vi "Drive Controller.vi"(8 "error in":errorcluster) -> ()   [LabVIEW 2017]
doc: "This VI executes continuously carrying out the current operation and responding to updates or new operation requests. It will often contain the timing or control code that is difficult to place directly in TeleOp. This VI generally opens all sensors and motors and isolates the rest of the robot code from knowing implementation details of how the operations are carried out."
uses:
  <vilib>/Rock Robotics/WPI/Framework/Completion Status.ctl
  Drive Setpoints.ctl
  Drive Operations.ctl
  <vilib>/Rock Robotics/WPI/SafetyOutput/WPI_SafetyOutputConfigMenu.ctl
  Motor Settings.ctl
  <vilib>/Rock Robotics/SystemInterfaces/DIO/FPGA_DIOPWMChannel.ctl
  <vilib>/Rock Robotics/SystemInterfaces/DIO/FPGA_DIOChannel.ctl
  <vilib>/Rock Robotics/WPI/Counter/WPI_CounterDigitalInputToDigitalSource.vi
  <vilib>/Rock Robotics/Network Tables/NT Write Boolean.vi
panel:
  in  "Interactive Values":T1
  in  "Buttons":cluster{"Execute Cmd":bool, "Abort Cmd":bool}
  out "Command Timing":cluster{"Start Time (ms)":u32, "Iterations":i32}
  out "Status":T3
  out "Setpoints":T4(graph)
  out "Current\nCmd":string
  # "Tip: The graph shows the motor setpoints. It may also be helpful to observe inputs and sensor values.\nYou may also want to display tuning or debugging controls."
  # "Interactive Command: You may fill in the settings for a command\nand schedule it with the Execute button. You can observe and abort\nany command while fine tuning the code for the controller."
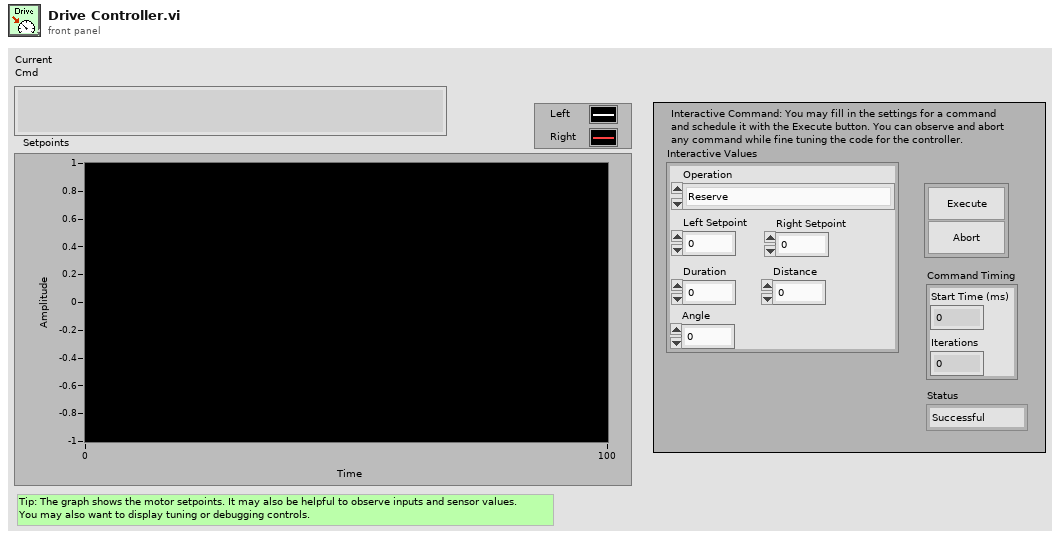
[diagram p1: front panel]
types:
  T1 = typedef "Drive Setpoints.ctl" = cluster{"Operation":T2, "Left Setpoint":dbl, "Right Setpoint":dbl, "Duration":dbl, "Distance":dbl, "Angle":dbl}
  T2 = typedef "Drive Operations.ctl" = enum16{"Reserve", "Read Current", "Immediate", "Drive for Angle", "Drive for Time", "Drive for Distance"}
  T3 = typedef "Completion Status.ctl" = enum16{"Successful", "Aborted", "Incomplete"}
  T4 = cluster{"Left Setpoint":dbl, "Right Setpoint":dbl}
  T5 = typedef "FPGA_DIOChannel.ctl" = enum8{"DIO 0", "DIO 1", "DIO 2", "DIO 3", "DIO 4", "DIO 5", "DIO 6", "DIO 7", "DIO 8", "DIO 9", "DIO MXP 0", "DIO MXP 1", "DIO MXP 2", "DIO MXP 3", "DIO MXP 4", "DIO MXP 5", "DIO MXP 6", "DIO MXP 7", "DIO MXP 8", "DIO MXP 9", "DIO MXP 10", "DIO MXP 11", "DIO MXP 12", "DIO MXP 13", "DIO MXP 14", "DIO MXP 15", "SPI Port CS1", "SPI Port CS2", "SPI Port CS3", "SPI Port MISO", "SPI Port MOSI", "Invalid"}
  T6 = typedef "Motor Settings.ctl" = cluster{"Rear Left Motor":cluster{"Inversion":bool, "PWM Channel":T7}, "Middle Left Motor":cluster{"Inversion":bool, "PWM Channel":T7}, "Front Left Motor":cluster{"Inversion":bool, "PWM Channel":T7}, "Rear Right Motor":cluster{"Inversion":bool, "PWM Channel":T7}, "Middle Right Motor":cluster{"Inversion":bool, "PWM Channel":T7}, "Front Right Motor":cluster{"Inversion":bool, "PWM Channel":T7}}
  T7 = typedef "FPGA_DIOPWMChannel.ctl" = enum8{"PWM 0", "PWM 1", "PWM 2", "PWM 3", "PWM 4", "PWM 5", "PWM 6", "PWM 7", "PWM 8", "PWM 9", "PWM MXP 0", "PWM MXP 1", "PWM MXP 2", "PWM MXP 3", "PWM MXP 4", "PWM MXP 5", "PWM MXP 6", "PWM MXP 7", "PWM MXP 8", "PWM MXP 9", "Invalid"}
  T8 = typedef "WPI_SafetyOutputConfigMenu.ctl" = enum16{"Enable", "Disable"}
  T9 = typedef "WPI_RobotDriveDevRef.ctl" = cluster{"DevStatus":errorcluster, "Motors[]":T10[], "Square Inputs":bool, "Max Output":dbl}
  T10 = typedef "WPI_MotorControlDeviceRef.ctl" = cluster{"DeviceStatus":errorcluster, "Type":T11, "PWM":cluster{"PWM Channel":T7, "DeadBand":T12}, "CAN":cluster{"Device Number":u8, "SetOutput VI Ref":variant, "GetOutput VI Ref":variant, "Enable VI Ref":variant, "Disable VI Ref":variant, "Data":variant}, "Invert":bool, "DIO PWM":cluster{"PWM \"Enable\" Channel":T7, "DIOChannel":T5, "PWM Rate":dbl}}
  T11 = typedef "WPI_MotorControlType.ctl" = enum16{"PWM", "CAN", "DIO PWM"}
  T12 = typedef "WPI_PWMDeadband.ctl" = cluster{"Name":string, "maxPositivePwm":i32, "minPositivePwm":i32, "centerPwm":i32, "maxNegativePwm":i32, "minNegativePwm":i32, "angularRange":u16}
  T13 = typedef "WPI_DigitalInputDevRef.ctl" = cluster{"DevStatus":errorcluster, "DIO Channel":T5}
  T14 = typedef "FPGA_CounterEncoderSourceConvertionLVSourceType.ctl" = cluster{"DevStatus":errorcluster, "AnalogTriggerMode?":bool, "DigitalMode":cluster{"DIO Channel":T15}, "AnalogTriggerMode":cluster{"AnalogTriggerIndex":T16, "OutputType":T17}}
  T15 = typedef "FPGA_DIODigitalSourceChannel.ctl" = enum8{"DIO 0", "DIO 1", "DIO 2", "DIO 3", "DIO 4", "DIO 5", "DIO 6", "DIO 7", "DIO 8", "DIO 9", "DIO MXP 0", "DIO MXP 1", "DIO MXP 2", "DIO MXP 3", "DIO MXP 4", "DIO MXP 5", "DIO MXP 6", "DIO MXP 7", "DIO MXP 8", "DIO MXP 9", "DIO MXP 10", "DIO MXP 11", "DIO MXP 12", "DIO MXP 13", "DIO MXP 14", "DIO MXP 15", "Disabled"}
  T16 = typedef "FPGA_AnalogTriggerIndex.ctl" = enum8{"Trig 0", "Trig 1", "Trig 2", "Trig 3", "Trig 4", "Trig 5", "Trig 6", "Trig 7", "Invalid"}
  T17 = typedef "FPGA_AnalogTriggerOutType.ctl" = enum16{"InWindow", "TriggerState", "Rising", "Falling"}
  T18 = typedef "WPI_EncoderDevRef.ctl" = cluster{"DevStatus":errorcluster, "EncoderIndex":T19, "CounterIndex":T20, "DistancePerCount":dbl, "Decoding Type":T21}
  T19 = typedef "FPGA_EncoderIdx.ctl" = enum8{"Enc 0", "Enc 1", "Enc 2", "Enc 3", "Enc 4", "Enc 5", "Enc 6", "Enc 7", "Invalid"}
  T20 = typedef "FPGA_CounterCtrSystemIndex.ctl" = enum8{"Ctr 0", "Ctr 1", "Ctr 2", "Ctr 3", "Ctr 4", "Ctr 5", "Ctr 6", "Ctr 7", "Invalid"}
  T21 = typedef "WPI_EncoderType.ctl" = enum16{"1x", "2x", "4x"}
  T22 = typedef "Command Status Info.ctl" = cluster{"Name":string, "Status":T3, "notifier out":T23}
  T23 = typedef "Completion Notifier.ctl" = refnum<notifier>
  T24 = cluster{"SubSystem Data":T1, cluster{"Start Time (ms)":u32, "Iterations":i32}, cluster{"Command Info":T22, "Description":string, "Default Command":T1, "queue out":refnum<queue>, "Subsystem Name":string}}
  T25 = cluster{"Yaw":dbl, "Roll":dbl, "Pitch":dbl, "Heading":dbl, "Fused Heading":dbl}
  T26 = cluster{"SubSystem Data":T1, cluster{"Start Time (ms)":u32, "Iterations":i32}, "Default Command Arguments":cluster{"Command Info":T22, "Description":string, "Default Command":T1, "queue out":refnum<queue>, "Subsystem Name":string}}
  T27 = cluster{"Don't move motors while reserved":dbl, "Don't move motors while reserved":dbl}
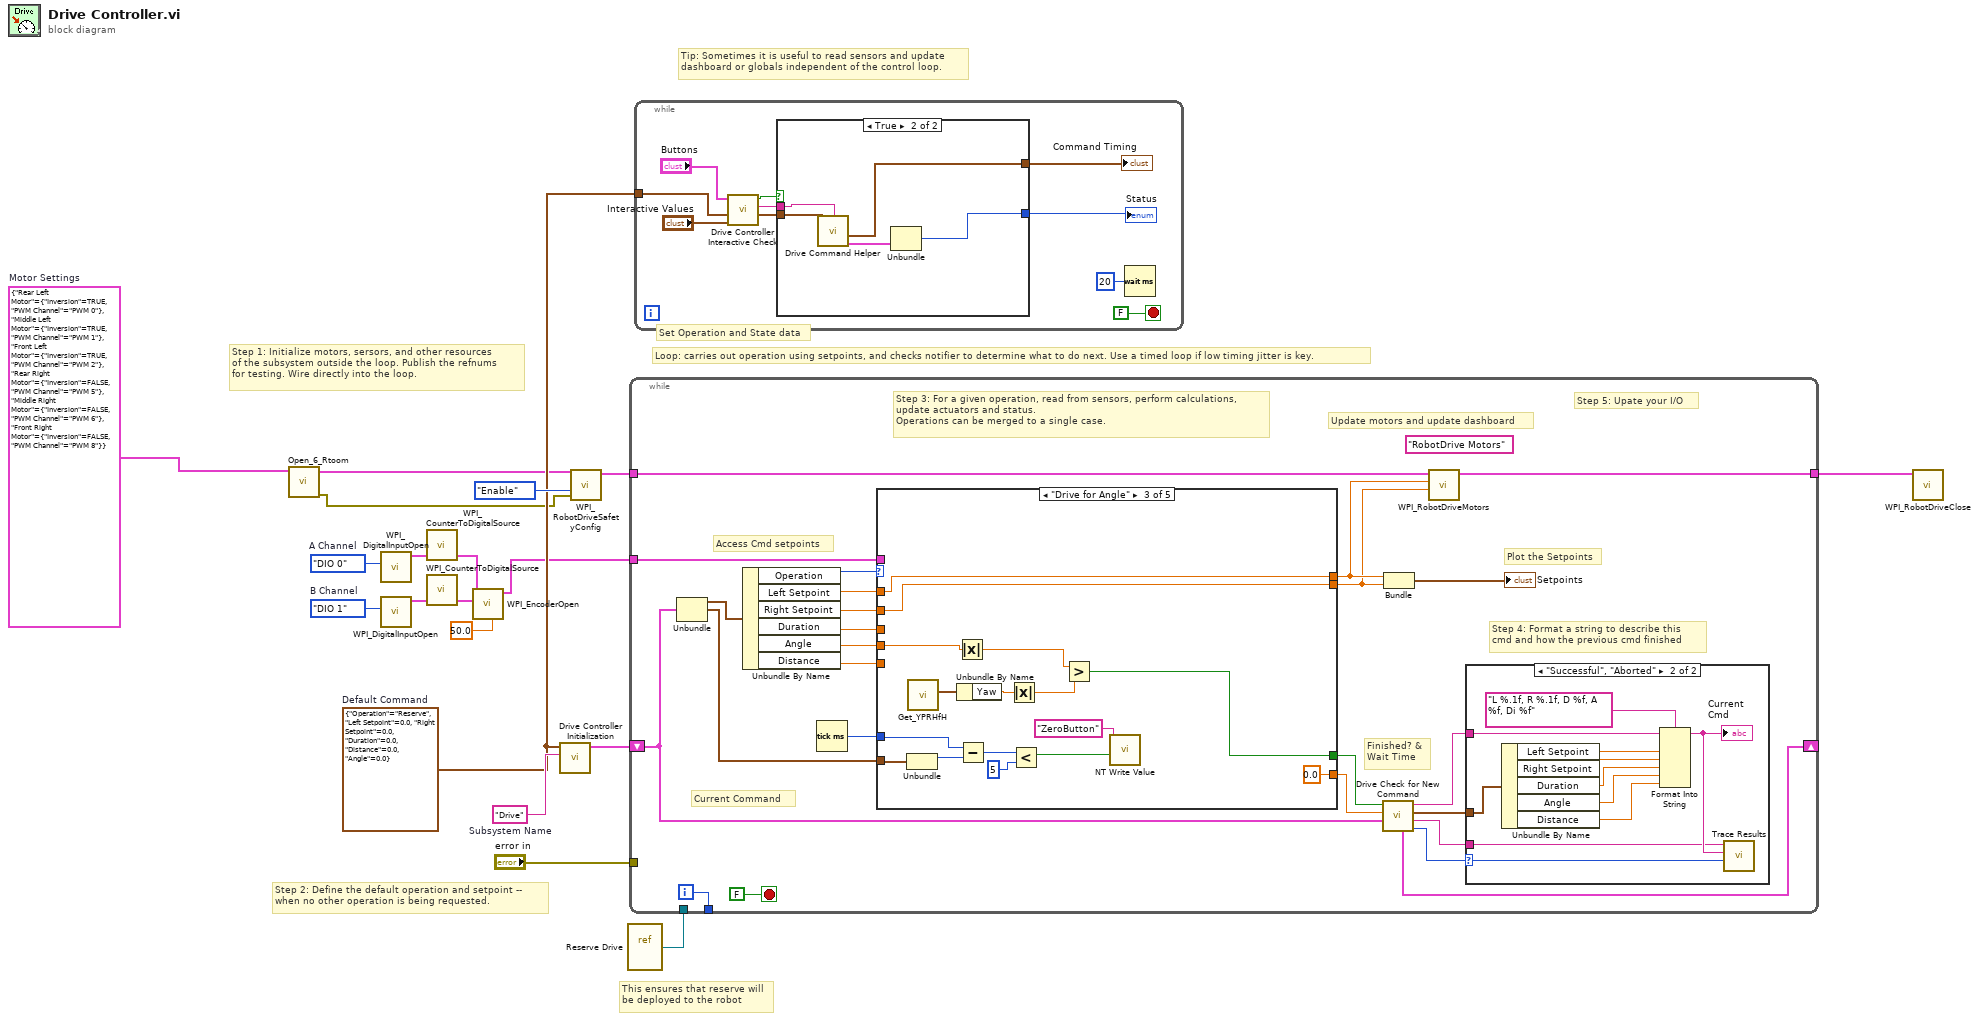
[diagram p0: block diagram]
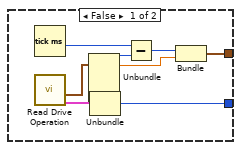
[diagram p2: hidden frame]
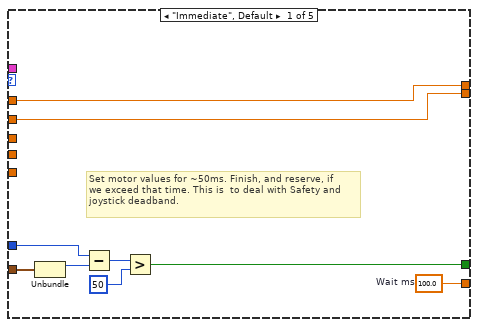
[diagram p4: hidden frame]
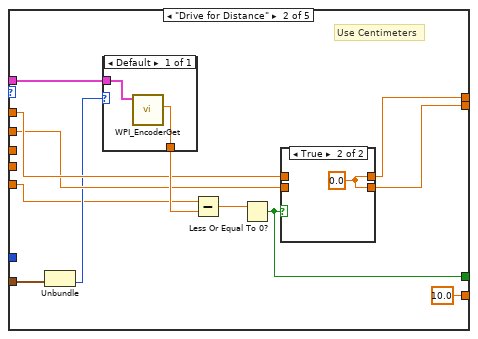
[diagram p5: hidden frame]
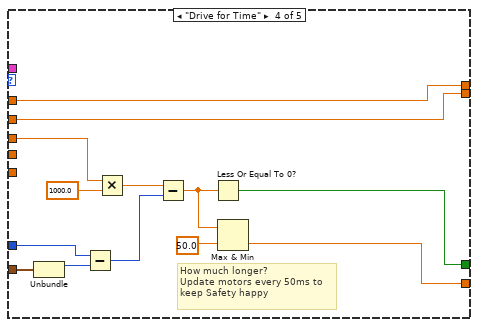
[diagram p7: hidden frame]
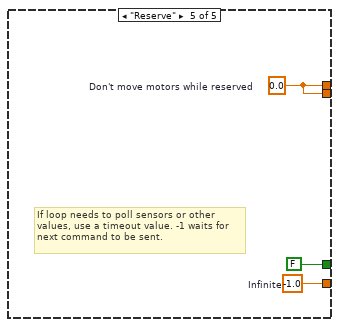
[diagram p8: hidden frame]
diagram:
  w4 = FPGA_DIOChannel."DIO 1"  # B Channel
  w3 = FPGA_DIOChannel."DIO 0"  # A Channel
  w9 = T6 {"Rear Left Motor"={"Inversion"=TRUE, "PWM Channel"=enum."PWM 0"}, "Middle Left Motor"={"Inversion"=TRUE, "PWM Channel"=enum."PWM 1"}, "Front Left Motor"={"Inversion"=TRUE, "PWM Channel"=enum."PWM 2"}, "Rear Right Motor"={"Inversion"=FALSE, "PWM Channel"=enum."PWM 5"}, "Middle Right Motor"={"Inversion"=FALSE, "PWM Channel"=enum."PWM 6"}, "Front Right Motor"={"Inversion"=FALSE, "PWM Channel"=enum."PWM 8"}}  # Motor Settings
  w13 = T1 {"Operation"=enum."Reserve", "Left Setpoint"=0.0, "Right Setpoint"=0.0, "Duration"=0.0, "Distance"=0.0, "Angle"=0.0}  # Default Command
  w19 = "Drive"  # Subsystem Name
  # "Set Operation and State data"
  # "This ensures that reserve will\nbe deployed to the robot"
  # "Tip: Sometimes it is useful to read sensors and update\ndashboard or globals independent of the control loop."
  # "Step 2: Define the default operation and setpoint --\nwhen no other operation is being requested."
  # "Step 1: Initialize motors, sersors, and other resources\nof the subsystem outside the loop. Publish the refnums\nfor testing. Wire directly into the loop."
  # "Loop: carries out operation using setpoints, and checks notifier to determine what to do next. Use a timed loop if low timing jitter is key."
  n1 = call "Open_6_Rtoom.vi"("Motor Settings"=w9) -> ("error out"=w10:errorcluster, "RobotDriveDevRef"=w11:T9)  [unwired: 8 in]
  n2 = call <vilib>:"WPI_DigitalInputOpen.vi"("DIO Channel"=w3) -> ("DigitalInputDevRef"=w7:T13)  [unwired: 1 in, 9 out]
  n3 = call <vilib>:"WPI_DigitalInputOpen.vi"("DIO Channel"=w4) -> ("DigitalInputDevRef"=w6:T13)  [unwired: 1 in, 9 out]
  n4 = call-poly <vilib>:"WPI_CounterToDigitalSource.vi"("DigitalInputDevRef"=w7) -> ("Digital Source"=w8:T14)  [unwired: 6 out]
  n5 = call-poly <vilib>:"WPI_CounterToDigitalSource.vi"("DigitalInputDevRef"=w6) -> ("Digital Source"=w5:T14)  [unwired: 6 out]
  n6 = call <vilib>:"WPI_EncoderOpen.vi"("DistancePerCount"=50.0, "BSource"=w5, "ASource"=w8) -> ("EncoderDevRef"=w1:T18)  [unwired: 5 in, 3 out]
  n7 = call "Drive Controller Initialization.vi"("Subsystem Name"=w19, "Default Command"=w13) -> ("Current Command"=w15:T24)  [unwired: 9 in]
  n8 = call <vilib>:"WPI_RobotDriveSafetyConfig.vi"("error in (no error)"=w10, "mode"=WPI_SafetyOutputConfigMenu."Enable", "RobotDriveDevRef"=w11) -> ("RobotDriveDevRef"=w17:T9)  [unwired: 7 in, 1 out]
  n9 = vi-ref "Reserve Drive.vi"() -> (w14:refnum<vi>)
  n10 = while {
    shift-right: [w31] -> _
    shift-left: w15 -> [w24]
    tunnel: [w43] -> _
    tunnel: w17 -> [w39]
    tunnel: "error in" -> [_]
    tunnel: w14 -> [_]
    tunnel: [w23] -> w12
    tunnel: w1 -> [w20]
    i -> [w43]
    stop <- FALSE stop-if-true
    (unwired) "RobotDrive Motors" ("Name")
    # "Step 5: Upate your I/O"
    # "Step 4: Format a string to describe this\ncmd and how the previous cmd finished"
    # "Current Command"
    # "Update motors and update dashboard"
    # "Plot the Setpoints"
    # "Access Cmd setpoints"
    # "Finished? &\nWait Time"
    # "Step 3: For a given operation, read from sensors, perform calculations,\nupdate actuators and status.\nOperations can be merged to a single case."
    n11 = Unbundle(w24) -> ("SubSystem Data"=w38:T1, w25:cluster{"Start Time (ms)":u32, "Iterations":i32})  [unwired: 1 out]
    n12 = Unbundle By Name(w38) -> ("Operation"=w37:T2, "Left Setpoint"=w36:dbl, "Right Setpoint"=w35:dbl, "Duration"=w34:dbl, "Angle"=w22:dbl, "Distance"=w21:dbl)
    n13 = Tick Count (ms)() -> (millisecond timer value=w33:u32)
    n14 = case shown="\"Drive for Angle\"" w37 {
      tunnel: [w64 10.0 ("Infinite") 0.0 ("Infinite") w98 w113] -> w30
      tunnel: [w57 w69 w84 w105 FALSE ("ignore previous (F)")] -> w29
      tunnel: w25 -> [w56 w67 w87 w107 _]
      tunnel: [w63 w72 w95 w104 w111] -> w41
      tunnel: [w62 w70 w96 w103 w111] -> w40
      tunnel: w36 -> [w63 w73 w95 w104 _]
      tunnel: w35 -> [w62 w71 w96 w103 _]
      tunnel: w34 -> [_ _ _ w102 _]
      tunnel: w33 -> [w58 _ w88 w101 _]
      tunnel: w22 -> [_ _ w94 _ _]
      tunnel: w21 -> [_ w65 _ _ _]
      tunnel: w20 -> [_ w76 _ _ _]
      frame "Immediate", Default {
        w64 = 100.0  # Wait ms
        # "Set motor values for ~50ms. Finish, and reserve, if\nwe exceed that time. This is  to deal with Safety and\njoystick deadband."
        n15 = Unbundle(w56) -> ("Start Time (ms)"=w59:u32)  [unwired: 1 out]
        n16 = Subtract(x=w58, y=w59) -> (x-y=w60:u32)
        n17 = Greater?(x=w60, y=u8 50 ("Left Motor")) -> (0:w57:bool)
      }
      frame "Drive for Distance" {
        # "Use Centimeters"
        n18 = Unbundle(w67) -> ("Iterations"=w66:i32)  [unwired: 1 out]
        n19 = case shown="Default" w66 {
          tunnel: w76 -> [w81]
          tunnel: [w80] -> w75
          frame Default {
            n20 = call <vilib>:"WPI_EncoderGet.vi"("EncoderDevRef"=w81) -> ("Distance"=w80:dbl)  [unwired: 5 in, 5 out]
          }
        }
        n21 = Subtract(x=w65, y=w75) -> (x-y=w74:dbl)
        n22 = Less Or Equal To 0?(x=w74) -> (x <= 0?=w69:bool)
        n23 = case shown="True" w69 {
          tunnel: w73 -> [w78 _]
          tunnel: [w78 w79] -> w72
          tunnel: w71 -> [w77 _]
          tunnel: [w77 w79] -> w70
          frame False {
          }
          frame True {
            w79 = 0.0 ("Left Setpoint")
          }
        }
      }
      frame "Drive for Angle" {
        n24 = Unbundle(w87) -> ("Start Time (ms)"=w89:u32)  [unwired: 1 out]
        n25 = call <vilib>:"Get_YPRHfH.vi"() -> ("YRPHfH"=w93:T25)  [unwired: 11 in]
        n26 = Absolute Value(x=w94) -> (abs(x)=w90:dbl)
        n27 = Unbundle By Name(w93) -> ("Yaw"=w92:dbl)
        n28 = Subtract(x=w88, y=w89) -> (x-y=w86:u32)
        n29 = Absolute Value(x=w92) -> (abs(x)=w91:dbl)
        n30 = Less?(x=w86, y=u32 5) -> (x < y?=w83:bool)
        n31 = Greater?(x=w90, y=w91) -> (0:w84:bool)
        n32 = call-poly <vilib>:"NT Write Value.vi"("Boolean"=w83, "Name"="ZeroButton") -> ()  [unwired: 9 in, 1 out]
      }
      frame "Drive for Time" {
        # "How much longer?\nUpdate motors every 50ms to\nkeep Safety happy"
        n33 = Unbundle(w107) -> ("Start Time (ms)"=w106:u32)  [unwired: 1 out]
        n34 = Subtract(x=w101, y=w106) -> (x-y=w110:u32)
        n35 = Multiply(x=w102, y=1000.0) -> (x*y=w109:dbl)
        n36 = Subtract(x=w109, y=w110) -> (x-y=w100:dbl)
        n37 = Less Or Equal To 0?(x=w100) -> (x <= 0?=w105:bool)
        n38 = Max & Min(x=w100, y=50.0) -> (min(x,y)=w98:dbl)  [unwired: 1 out]
      }
      frame "Reserve" {
        w111 = 0.0  # Don't move motors while reserved
        w113 = -1.0  # Infinite
        # "If loop needs to poll sensors or other\nvalues, use a timeout value. -1 waits for\nnext command to be sent."
      }
    }
    n39 = call "Drive Check for New Command.vi"("input cluster"=w24, "Wait time (ms)"=w30, "Finished?"=w29) -> ("Completion"=w32:T3, "Subsystem Name"=w26:string, "Current Command"=w27:T1, "Initial Trace String"=w28:string, "Next Command"=w31:T26)  [unwired: 4 in]
    n40 = Bundle("Don't move motors while reserved"=w41, "Don't move motors while reserved"=w40) -> (→"Setpoints":T27)  [unwired: 1 in]
    n41 = call <vilib>:"WPI_RobotDriveMotors.vi"("RightSpeed"=w40, "LeftSpeed"=w41, "RobotDriveDevRef"=w39) -> ("RobotDriveDevRef"=w23:T9)  [unwired: 1 in, 7 out]
    n42 = case shown="\"Successful\", \"Aborted\"" w32 {
      selector: w32 -> [_ w55]
      tunnel: w28 -> [_ w50]
      tunnel: w27 -> [_ w51]
      tunnel: w26 -> [_ w47]
      frame "Incomplete", Default {
        # "Continuing current command"
      }
      frame "Successful", "Aborted" {
        # "Report and setup for next command"
        n43 = Unbundle By Name(w51) -> ("Left Setpoint"=w53:dbl, "Right Setpoint"=w54:dbl, "Duration"=w48:dbl, "Angle"=w46:dbl, "Distance"=w45:dbl)
        n44 = Format Into String(format string="L %.1f, R %.1f, D %f, A %f, Di %f", initial string=w50, w53, w54, w48, w46, w45) -> (resulting string=w49:string)  [unwired: 1 in, 1 out]
        "Current\nCmd" <- w49
        n45 = call <vilib>:"Trace Results.vi"("Status of previous command"=w55, "Description"=w49, "Subsystem"=w47) -> ()  [unwired: 9 in]
      }
    }
  }
  n46 = while {
    tunnel: w13 -> [w115]
    stop <- FALSE stop-if-true
    n47 = call "Drive Controller Interactive Check.vi"("Interactive Command In"="Interactive Values", "Default Command"=w115, "Buttons"="Buttons") -> ("Interactive Command Out"=w117:T1, "Trace String"=w118:string, "Schedule"=w119:bool)  [unwired: 6 in]
    n48 = case shown="True" w119 {
      tunnel: [w128 w136] -> w120
      tunnel: [w127 w132] -> w121
      tunnel: w118 -> [_ w134]
      tunnel: w117 -> [_ w133]
      frame False {
        n49 = Tick Count (ms)() -> (millisecond timer value=w131:u32)
        n50 = call "Read Drive Operation.vi"() -> ("Command Info"=w125:T22, "SubSystem Data"=w124:T1)  [unwired: 9 in, 1 out]
        n51 = Unbundle(w124) -> ("Operation"=w129:T2, "Left Setpoint"=w126:dbl)  [unwired: 4 out]
        n52 = Unbundle(w125) -> ("Status"=w128:T3)  [unwired: 2 out]
        n53 = Subtract(x=w131, y=w129) -> (x-y=w130:u32)
        n54 = Bundle(w130, "Left Setpoint"=w126) -> (w127:cluster{u32, "Left Setpoint":dbl})  [unwired: 1 in]
      }
      frame True {
        n55 = call "Drive Command Helper.vi"("Description"=w134, "SubSystem Data"=w133) -> ("Command Info Out"=w135:T22, "Command Timing"=w132:cluster{"Start Time (ms)":u32, "Iterations":i32})  [unwired: 7 in, 1 out]
        n56 = Unbundle(w135) -> ("Status"=w136:T3)  [unwired: 2 out]
      }
    }
    "Status" <- w120
    "Command Timing" <- w121
    n57 = Wait (ms)(milliseconds to wait=u32 20) -> ()  [unwired: 1 out]
  }
  n58 = call <vilib>:"WPI_RobotDriveClose.vi"("RobotDriveDevRef"=w12) -> ()  [unwired: 10 in, 1 out]
